vi "Monitor-ZoomCenterPosition.vi"(11 "Zoom rect coords":T1) -> (3 "Zoom Center Coord":cluster{" X":dbl, "Y":dbl})   [LabVIEW 2016]
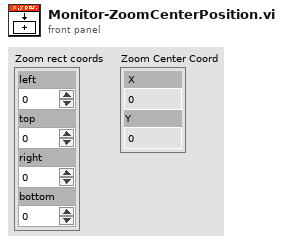
[diagram p1: front panel]
types:
  T1 = cluster{"left":i16, "top":i16, "right":i16, "bottom":i16}
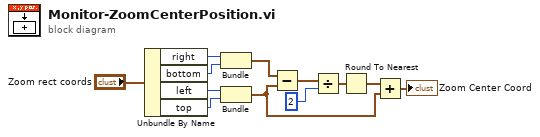
[diagram p0: block diagram]
diagram:
  n1 = Unbundle By Name("Zoom rect coords") -> ("right"=w11:i16, "bottom"=w2:i16, "left"=w1:i16, "top"=w10:i16)
  n2 = Bundle("right"=w11, "bottom"=w2) -> (w9:cluster{"right":i16, "bottom":i16})  [unwired: 1 in]
  n3 = Bundle("left"=w1, "top"=w10) -> (w4:cluster{"left":i16, "top":i16})  [unwired: 1 in]
  n4 = Subtract ("Height")(x=w9, y=w4) -> (x-y=w8:cluster{i16, i16})
  n5 = Divide(x=w8, y=i16 2) -> (x/y=w6:cluster{dbl, dbl})
  n6 = Round To Nearest(number=w6) -> (nearest integer value=w5:cluster{dbl, dbl})
  n7 = Add(x=w5, y=w4) -> (x+y=→"Zoom Center Coord":cluster{dbl, dbl})
